vi "Set Initialization Data - System Monitor UI.vi"(8 "error in":errorcluster, 11 "Host NI 9205 Demo in":refnum<class "Host NI 9205 Demo.lvclass">) -> (0 "error out":errorcluster, 3 "Host NI 9205 Demo out":refnum<class "Host NI 9205 Demo.lvclass">)   [LabVIEW 2017, in "Host NI 9205 Demo.lvclass"]
doc: "In this VI you can set the initialization data of a statically-linked subWorker."
uses:
  Host NI 9205 Demo.lvclass
  System Monitor UI/Initialization Data.ctl
  System Monitor UI/Response Cases.ctl
  Host NI 9205 Demo.lvclass/Host NI 9205 Demo.ctl
  System Monitor UI/System Monitor UI.lvclass
  C:/Program Files (x86)/National Instruments/LabVIEW 2017/vi.lib/addons/_Workers/Library/Classes/Worker/Worker.lvclass
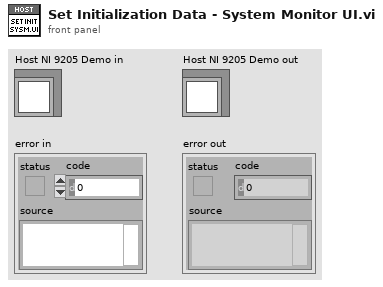
[diagram p1: front panel]
types:
  T1 = typedef "System Monitor UI.lvclass/Initialization Data.ctl" = cluster{"Response Cases":T2}
  T2 = typedef "System Monitor UI.lvclass/Response Cases.ctl" = cluster{"Placeholder - Can be deleted":string}
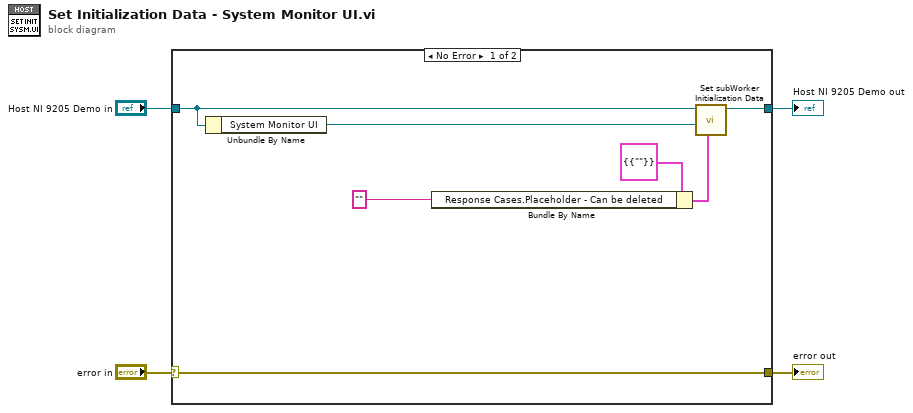
[diagram p0: block diagram]
diagram:
  n1 = case shown="No Error" "error in" {
    selector: "error in" -> [w11 w13]
    tunnel: [w11 w13] -> w3
    tunnel: [w9 w12] -> w2
    tunnel: "Host NI 9205 Demo in" -> [w8 w12]
    frame No Error {
      n2 = Unbundle By Name(w8) -> ("System Monitor UI"=w10:refnum<class "System Monitor UI.lvclass">)
      n3 = Bundle By Name(cluster=T1 {"Response Cases"={"Placeholder - Can be deleted"=""}} ("Initialization Data"), "Response Cases.Placeholder - Can be deleted"="" ("Placeholder")) -> (w6:T1)
      n4 = call-dynamic "Set subWorker Initialization Data.vi"("Initialization Data"=w6, "subWorker"=w10, "Worker"=w8) -> ("Worker out"=w9:refnum<class "Host NI 9205 Demo.lvclass">)  [unwired: 8 in]
    }
    frame Error {
    }
  }
  "error out" <- w3
  "Host NI 9205 Demo out" <- w2
